vi "Set_Data.vi"(1 "device name":tag="Dev0", 2 "error in":errorcluster, 3 "Data":u8, 4 "Ch":u8) -> (0 "error out":errorcluster)   [LabVIEW 2017]
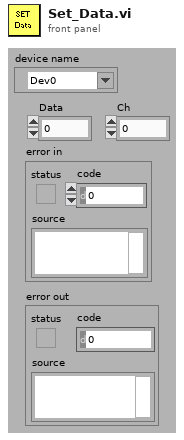
[diagram p1: front panel]
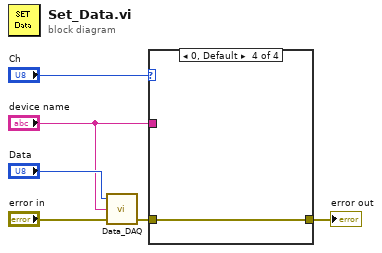
[diagram p0: block diagram]
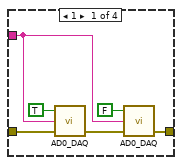
[diagram p2: hidden frame]
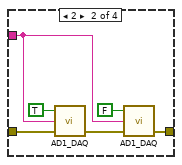
[diagram p3: hidden frame]
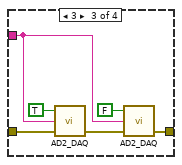
[diagram p4: hidden frame]
diagram:
  n1 = call "Data_DAQ.vi"("error in"="error in", "device name"="device name", "Input"="Data") -> ("error out"=w2:errorcluster)  [unwired: 2 in]
  n2 = case shown="0, Default" "Ch" {
    tunnel: [w9 w15 w22 w25] -> w5
    tunnel: w2 -> [w8 w14 w20 w25]
    tunnel: "device name" -> [w7 w13 w19 _]
    frame 1 {
      n3 = call "AD0_DAQ.vi"("error in"=w8, "device name"=w7, "Boolean In"=TRUE) -> ("error out"=w10:errorcluster)  [unwired: 2 in]
      n4 = call "AD0_DAQ.vi"("error in"=w10, "device name"=w7, "Boolean In"=FALSE) -> ("error out"=w9:errorcluster)  [unwired: 2 in]
    }
    frame 2 {
      n5 = call "AD1_DAQ.vi"("error in"=w14, "device name"=w13, "Boolean In"=TRUE) -> ("error out"=w16:errorcluster)  [unwired: 2 in]
      n6 = call "AD1_DAQ.vi"("error in"=w16, "device name"=w13, "Boolean In"=FALSE) -> ("error out"=w15:errorcluster)  [unwired: 2 in]
    }
    frame 3 {
      n7 = call "AD2_DAQ.vi"("error in"=w20, "device name"=w19, "Boolean In"=TRUE) -> ("error out"=w23:errorcluster)  [unwired: 2 in]
      n8 = call "AD2_DAQ.vi"("error in"=w23, "device name"=w19, "Boolean In"=FALSE) -> ("error out"=w22:errorcluster)  [unwired: 2 in]
    }
    frame 0, Default {
    }
  }
  "error out" <- w5
